vi "get_discont_step_size_float.vi"(9 "current pixel (iteration)":i32, 11 "current row in image":dbl[](array[numeric])) -> (3 "step_size":dbl)   [LabVIEW 2011]
doc: "Calculates the step size between the two pixels of a discontinuity. The step size is calulated by the difference between the two pixels plus an average slope, calculate as the average slope before and after the discontinuity."
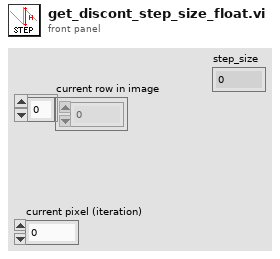
[diagram p1: front panel]
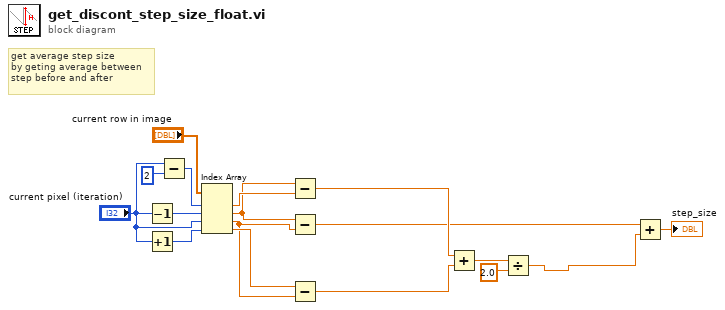
[diagram p0: block diagram]
diagram:
  # "get average step size\nby geting average between\nstep before and after"
  n1 = Decrement(x="current pixel (iteration)") -> (x-1=w10:i32)
  n2 = Increment(x="current pixel (iteration)") -> (x+1=w9:i32)
  n3 = Subtract(x="current pixel (iteration)", y=2) -> (x-y=w11:i32)
  n4 = Index Array(array="current row in image", index #1=w11, index #2=w10, index #3="current pixel (iteration)", index #4=w9) -> (element #1=w4:dbl, element #2=w2:dbl, element #3=w1:dbl, element #4=w3:dbl)
  n5 = Subtract(x=w2, y=w4) -> (x-y=w15:dbl)
  n6 = Subtract(x=w2, y=w1) -> (x-y=w7:dbl)
  n7 = Subtract(x=w3, y=w1) -> (x-y=w14:dbl)
  n8 = Add(x=w15, y=w14) -> (x+y=w16:dbl)
  n9 = Divide(x=w16, y=2.0) -> (x/y=w5:dbl)
  n10 = Add(x=w7, y=w5) -> (x+y=→"step_size":dbl)
